vi "Configure Immediate Trigger.vi"(0 "device session in":refnum<class "Device Session.lvclass">, 11 "error in":errorcluster) -> (4 "device session out":refnum<class "Device Session.lvclass">, 15 "error out":errorcluster)   [LabVIEW 2021, in "Device Session.lvclass"]
doc: "Configures the acquisition for an immediate software trigger.\n\n<B>Input Parameters</B>\n\n<B>device session in</B> is a reference to the Device Session object, which contains a session to each instrument design library used in this sample project. This parameter is obtained from the 'Open Session' VI.\n\n<B>error in</B> describes error conditions that occur before this node runs. This input provides standard 'error in' functionality.\n\n<B>Output Parameters</B>\n\n<B>device session out</B> passes a reference to the session to the next VI.\n\n<B>error out</B> contains error information. This output provides standard 'error out' functionality."
uses:
  Device Session.lvclass
  Device Session.lvclass/Device Session.ctl
  <vilib>/Utility/error.llb/Error Cluster From Error Code.vi
  <vilib>/rvi/errors/niLvFpgaAdjustHostInterfaceError.vi
  <vilib>/rvi/interface/nirviReadWriteControl/nirviReadWriteControl.xnode
  FPGA Refnum.ctl
  NiFpgaLv.dll
  <vilib>/rvi/interface/Simulation/niFpgaSimulationCallBeginRW.vi
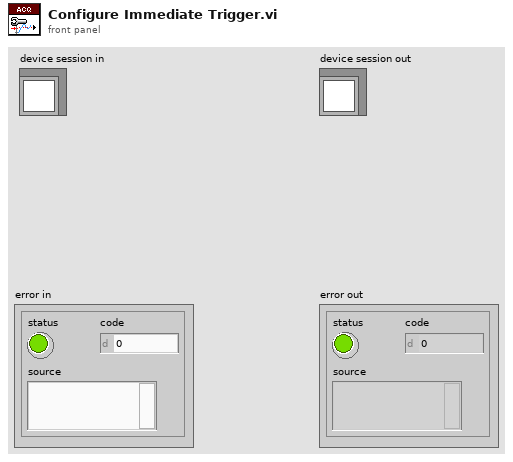
[diagram p1: front panel]
types:
  T1 = enum16{"Immediate", "A", "B", "OR", "AND", "A THEN B", "B THEN A", "High Resolution"}
  T2 = typedef "Device Session.lvclass/Device Session Object.ctl" = cluster{"fpga reference":T3, "reg bus":refnum<class "niInstr FIFO Register Bus v1 Host.lvclass">, "subsystem map":refnum<class "niInstr Subsystem Map v1 Host.lvclass">, "cal data":refnum<class "niHSAI Cal Data v1 Host.lvclass">, "config":refnum<class "niHSAI Group A Config v1 Host.lvclass">, "acquisition 0":refnum<class "niInstr Multirecord Acquisition v1 Host.lvclass">, "acquisition 1":refnum<class "niInstr Multirecord Acquisition v1 Host.lvclass">, "number of selected acq channels":u8, "selected acq channels":bool[], "number of channels":u32, "configured channels":bool[], "acq configuration":cluster{"number of samples":u64, "number of records":u64, "pretrigger samples":u64}, "actual channel configuration":T4[], "sample clock rate (Hz)":dbl, "scaling coefficients":T8[]}
  T3 = typedef "Device Session.lvclass/FPGA Refnum.ctl" = refnum<k20>
  T4 = typedef "niHSAI Types v1 Host.lvlib/Channel Configuration.ctl" = cluster{"channel":u32, "coupling":T5, "impedance":T6, "bandwidth":T7, "vertical range":dbl, "vertical offset":dbl}
  T5 = typedef "niHSAI Types v1 Host.lvlib/Coupling.ctl" = enum8{"Default", "DC", "AC"}
  T6 = typedef "niHSAI Types v1 Host.lvlib/Impedance.ctl" = enum8{"Default", "1 mega ohm", "50 ohm"}
  T7 = typedef "niHSAI Types v1 Host.lvlib/Bandwidth.ctl" = enum8{"Default", "Full Bandwidth", "Anti-alias Filter", "150 MHz"}
  T8 = typedef "niInstr Multirecord Acquisition v1 Host.lvclass/Scaling Coefficient.ctl" = cluster{"gain":dbl, "offset":dbl}
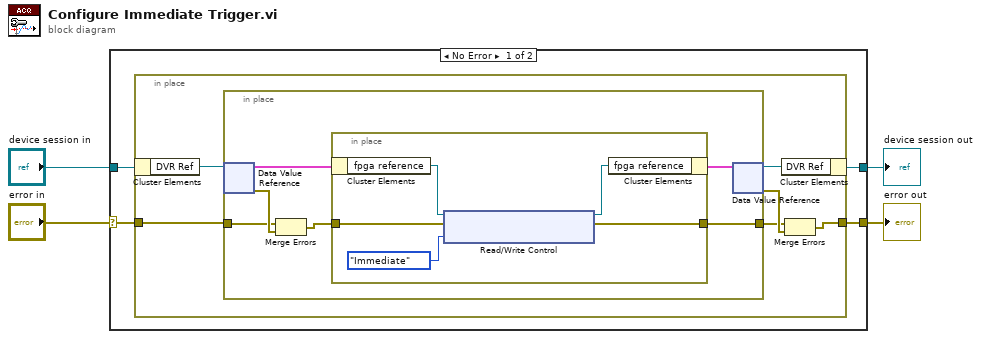
[diagram p0: block diagram]
diagram:
  n1 = case shown="No Error" "error in" {
    selector: "error in" -> [w8 w27]
    tunnel: "device session in" -> [w6 w26]
    tunnel: [w5 w26] -> w3
    tunnel: [w7 w27] -> w4
    frame No Error {
      n2 = in-place {
        in-place-border: w8 -> [w14]
        in-place-border: [w9] -> w7
        n3 = in-place-cluster #1(w6) -> ("DVR Ref"=w11:refnum<data-value>)
        n4 = in-place {
          in-place-border: w14 -> [w19]
          in-place-border: [w18] -> w12
          n5 = in-place-dvr #2(w11) -> (w16:T2, w20:errorcluster)
          n6 = Merge Errors(w19, w20) -> (w17:errorcluster)
          n7 = in-place {
            in-place-border: [w25] -> w18
            in-place-border: w17 -> [w23]
            n8 = in-place-cluster #3(w16) -> ("fpga reference"=w22:T3)
            n9 = xnode "Read/Write Control"("FPGA VI Reference In"=w22, "error in"=w23, "trigger.combination type"=T1."Immediate" ("trigger.combination.type")) -> ("FPGA VI Reference Out"=w21:T3, "error out"=w25:errorcluster)
            n10 = in-place-cluster #3("fpga reference"=w21) -> (w15:T2)
          }
          n11 = in-place-dvr #2(w15) -> (w10:refnum<data-value>, w13:errorcluster)
        }
        n12 = in-place-cluster #1("DVR Ref"=w10) -> (w5:refnum<class "Device Session.lvclass">)
        n13 = Merge Errors(w12, w13) -> (w9:errorcluster)
      }
    }
    frame Error {
    }
  }
  "error out" <- w4
  "device session out" <- w3
